vi "Reshape Move Array.vi"(10 "Profile in":dbl[](array[numeric])) -> (2 "Profile out":dbl[][](array[numeric]))   [LabVIEW 2013]
doc: "This sub-VI reshapes the position command array into a 2-dimensional array of tripplets comprising the\nXYZ commands per time step."
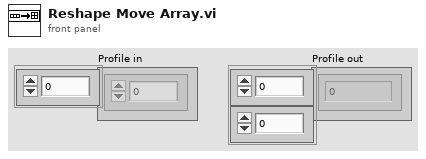
[diagram p1: front panel]
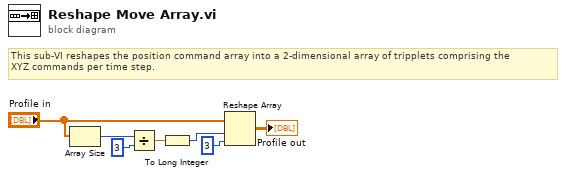
[diagram p0: block diagram]
diagram:
  # "This sub-VI reshapes the position command array into a 2-dimensional array of tripplets comprising the\nXYZ commands per time step."
  n1 = Array Size(array="Profile in") -> (size(s)=w5:i32)
  n2 = Divide(x=w5, y=3) -> (x/y=w3:dbl)
  n3 = To Long Integer(number=w3) -> (32bit integer=w1:i32)
  n4 = Reshape Array("Profile in", w1, 3 ("dimension size")) -> (→"Profile out":dbl[][])
